vi "Convert to GUI Event.vi"(4 "Event":T2={"Time Stamp"=timestamp(0 s since 1904-01-01), "Event Level"=enum."Info", "Context"="", "Message"="", "Error"={"status"=FALSE, "code"=0, "source"=""}}) -> (7 "Event Element":T1)   [LabVIEW 2020, in "Volatus.lvlib" / "Event Reporter Module.lvclass"]
uses:
  Event Reporter Module.lvclass
  Event.ctl
  Event Level.ctl
  Event Element.ctl
  Event Reporter Module.lvclass/Event Reporter Module.ctl
  Volatus.lvlib
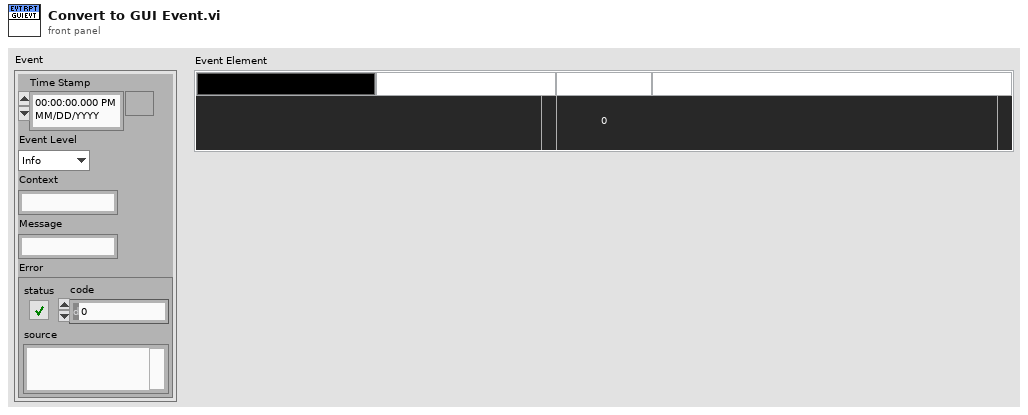
[diagram p1: front panel]
types:
  T1 = typedef "Volatus.lvlib/Event Reporter Module.lvclass/Event Element.ctl" = cluster{"Node":string, "Node Color":u32, "Timestamp":string, "TS Color":u32, "Level":string, "Level Color":u32, "Context":string, "Context Color":u32, "Message":string, "Error Code":i32, "Error Source":string}
  T2 = typedef "Volatus.lvlib/Event.ctl" = cluster{"Time Stamp":timestamp, "Event Level":T3, "Context":string, "Message":string, "Error":errorcluster}
  T3 = typedef "Volatus.lvlib/Event Level.ctl" = enum16{"Debug", "Info", "Warning", "Error"}
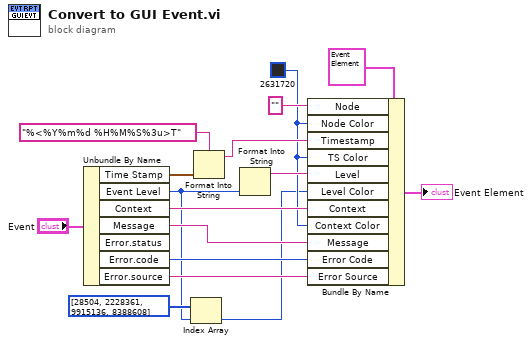
[diagram p0: block diagram]
diagram:
  w5 = u32 2631720 ("System Color")
  n1 = Unbundle By Name("Event") -> ("Time Stamp"=w14:timestamp, "Event Level"=w2:T3, "Context"=w8:string, "Message"=w7:string, "Error.code"=w12:i32, "Error.source"=w6:string)  [unwired: 1 out]
  n2 = Index Array(array=u32[] [28504, 2228361, 9915136, 8388608], index=w2) -> (element=w1:u32)
  n3 = Format Into String(format string="%<%Y%m%d %H%M%S%3u>T", w14) -> (resulting string=w11:string)  [unwired: 2 in, 1 out]
  n4 = Format Into String(w2) -> (resulting string=w9:string)  [unwired: 3 in, 1 out]
  n5 = Bundle By Name(cluster=T1 {"Node"="", "Node Color"=2631720, "Timestamp"="YYYYMMDD 000000.000", "TS Color"=2631720, "Level"="", "Level Color"=2631720, "Context"="", "Context Color"=2631720, "Message"="", "Error Code"=-2147483648, "Error Source"=""} ("Event Element"), "Node"="" ("System"), "Node Color"=w5, "Timestamp"=w11, "TS Color"=w5, "Level"=w9, "Level Color"=w1, "Context"=w8, "Context Color"=w5, "Message"=w7, "Error Code"=w12, "Error Source"=w6) -> (→"Event Element":T1)
